vi "Get Channel Indices.vi"(8 "error in (no error)":errorcluster, 11 "Control Experiment in":refnum<class "Control Experiment.lvclass">) -> (0 "error out":errorcluster, 2 "Indices":T1, 3 "Control Experiment out":refnum<class "Control Experiment.lvclass">)   [LabVIEW 2016, in "Control Experiment.lvclass"]
uses:
  Control Experiment.lvclass
  Control Experiment.lvclass/Control Experiment.ctl
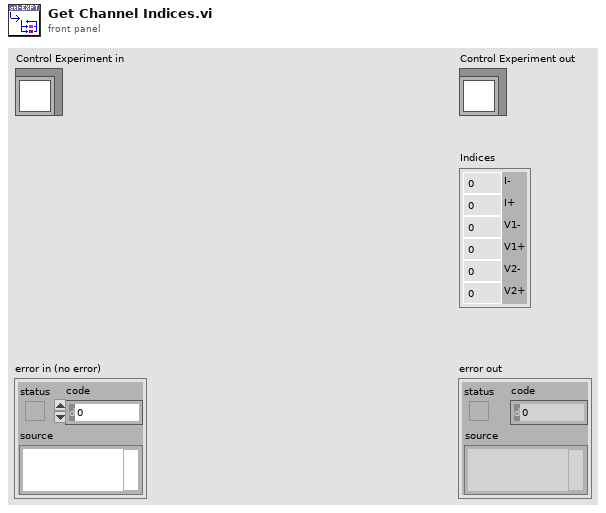
[diagram p1: front panel]
types:
  T1 = cluster{"I-":i32, "I+":i32, "V1-":i32, "V1+":i32, "V2-":i32, "V2+":i32}
  T2 = cluster{"[0]":i32, "[1]":i32, "[2]":i32, "[3]":i32, "[4]":i32, "[5]":i32}
  T3 = typedef "Dictionary Object RefNum__ogtk.ctl" = refnum<k1>
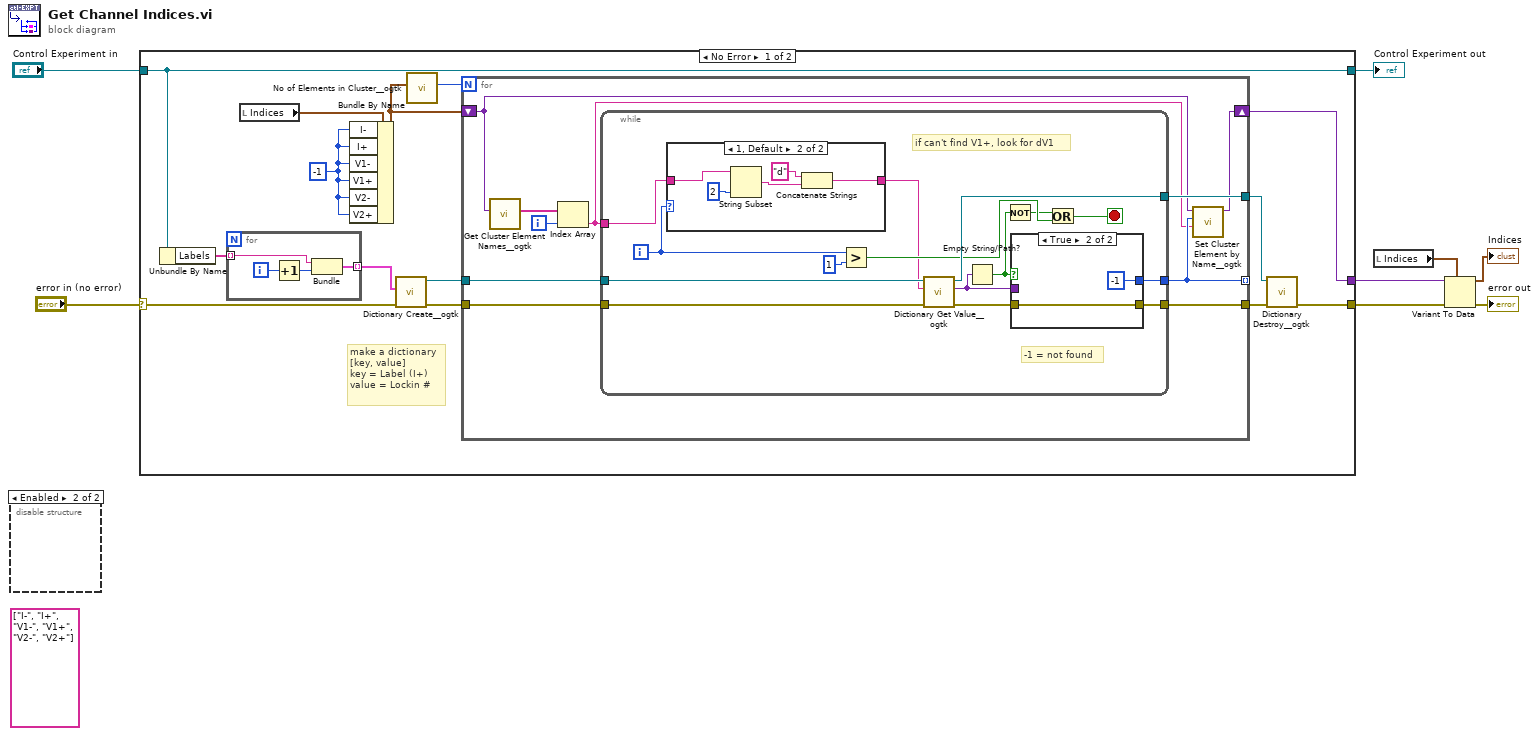
[diagram p0: block diagram]
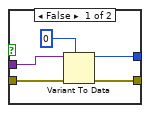
[diagram p3: hidden frame]
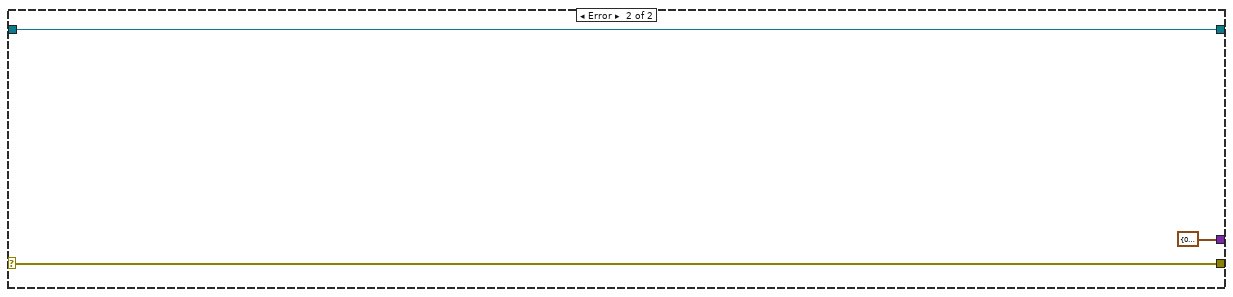
[diagram p4: hidden frame]
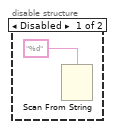
[diagram p5: hidden frame]
diagram:
  (unwired) string[] ["I-", "I+", "V1-", "V1+", "V2-", "V2+"]
  n1 = disable-structure shown="Enabled" {
    frame Disabled {
      n2 = Scan From String(format string="%d") -> ()  [unwired: 5 in, 3 out]
    }
    frame Enabled {
    }
  }
  n3 = case shown="No Error" "error in (no error)" {
    selector: "error in (no error)" -> [w22 w68]
    tunnel: [w17 w68] -> w2
    tunnel: [w14 w67] -> w6
    tunnel: "Control Experiment in" -> [w14 w67]
    tunnel: [w15 T2 {"[0]"=0, "[1]"=0, "[2]"=0, "[3]"=0, "[4]"=0, "[5]"=0}] -> w5
    frame No Error {
      w10 = -1 ("I-")
      # "make a dictionary\n[key, value]\nkey = Label (I+)\nvalue = Lockin #"
      n4 = Unbundle By Name(w14) -> ("Labels"=w16:string[])
      n5 = for {
        tunnel: w16 -> [w63] mode=indexing
        tunnel: [w65] -> w23 mode=indexing
        i -> [w64]
        n6 = Increment(x=w64) -> (x+1=w62:i32)
        n7 = Bundle("label"=w63, w62) -> (w65:cluster{"label":string, i32})  [unwired: 1 in]
      }
      n8 = local read "Indices"() -> (w12:T1)
      n9 = Bundle By Name(cluster=w12, "I-"=w10, "I+"=w10, "V1-"=w10, "V1+"=w10, "V2-"=w10, "V2+"=w10) -> (w11:T1)
      n10 = call <userlib>:"Dictionary Create__ogtk.vi"("error in (no error)"=w22, "initial dictionary (empty)"=w23) -> ("error out"=w18:errorcluster, "dictionary out"=w21:T3)  [unwired: 8 in]
      n11 = call <userlib>:"No of Elements in Cluster__ogtk.vi"("Cluster"=w11) -> ("Number of Elements"=w13:u16)  [unwired: 9 in, 1 out]
      n12 = for {
        N: w13 -> [_]
        tunnel: w21 -> [w33]
        tunnel: [w32] -> w20
        tunnel: w18 -> [w31]
        tunnel: [w25] -> w19
        tunnel: [w30] -> _ mode=indexing
        shift-right: [w26] -> w15
        shift-left: w11 -> [w29]
        i -> [w27]
        n13 = call <userlib>:"Get Cluster Element Names__ogtk.vi"("Cluster"=w29) -> ("Element Names"=w28:string[])  [unwired: 9 in, 1 out]
        n14 = Index Array(array=w28, index=w27) -> (element=w24:string)
        n15 = while {
          tunnel: [w45] -> w30
          tunnel: w24 -> [w35]
          tunnel: w33 -> [w48]
          tunnel: [w47] -> w32
          tunnel: w31 -> [w46]
          tunnel: [w43] -> w25
          i -> [w37]
          stop <- w41 stop-if-true
          # "-1 = not found"
          # "if can't find V1+, look for dV1"
          n16 = case shown="1, Default" w37 {
            tunnel: [w49 w52] -> w36
            tunnel: w35 -> [w49 w54]
            frame 0 {
            }
            frame 1, Default {
              n17 = String Subset(string=w54, length (rest)=2 ("length (rest)")) -> (substring=w51:string)  [unwired: 1 in]
              n18 = Concatenate Strings("d" ("string"), w51) -> (w52:string)
            }
          }
          n19 = Greater?(x=w37, y=1) -> (0:w38:bool)
          n20 = call <userlib>:"Dictionary Get Value__ogtk.vi"("error in"=w46, "key"=w36, "dictionary"=w48) -> ("error out"=w44:errorcluster, "value"=w42:variant, "dictionary out"=w47:T3)  [unwired: 5 in, 1 out]
          n21 = Empty String/Path?(string/path=w42) -> (empty?=w40:bool)
          n22 = Not(x=w40) -> (.not. x?=w34:bool)
          n23 = case shown="True" w40 {
            tunnel: [w59 w60] -> w43
            tunnel: [w58 -1 ("x+1")] -> w45
            tunnel: w42 -> [w57 _]
            tunnel: w44 -> [w55 w60]
            frame False {
              n24 = Variant To Data(error in=w55, type=0 ("x+1"), Variant=w57) -> (data=w58:i32, error out=w59:errorcluster)
            }
            frame True {
            }
          }
          n25 = Or(x=w34, y=w38) -> (x .or. y?=w41:bool)
        }
        n26 = call <userlib>:"Set Cluster Element by Name__ogtk.vi"("Element Name (\"\": New Element Data Name)"=w24, "New Element Value"=w30, "Cluster"=w29) -> ("VCluster out"=w26:variant)  [unwired: 6 in, 2 out]
      }
      n27 = call <userlib>:"Dictionary Destroy__ogtk.vi"("error in (no error)"=w19, "dictionary"=w20) -> ("error out"=w17:errorcluster)  [unwired: 9 in]
    }
    frame Error {
    }
  }
  "Control Experiment out" <- w6
  n28 = local read "Indices"() -> (w4:T1)
  n29 = Variant To Data(error in=w2, type=w4, Variant=w5) -> (data=→"Indices":T1, error out=→"error out":errorcluster)
